vi "isEnd.vi"(10 "pos":i32[][](array[numeric]), 11 "exist":i32[][](array[numeric])) -> (3 "isEnd":i16)   [LabVIEW 2022 SP3, in "subvis.lvlib"]
uses:
  subvis.lvlib
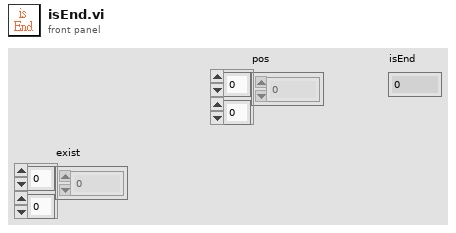
[diagram p1: front panel]
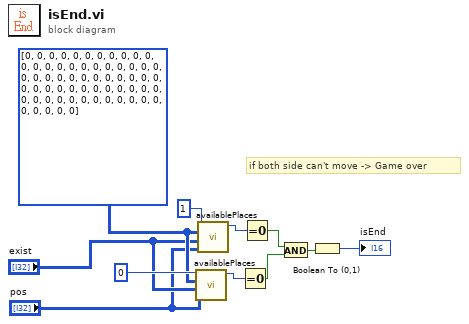
[diagram p0: block diagram]
diagram:
  w4 = i32[][] [[0, 0, 0, 0, 0, 0, 0, 0], [0, 0, 0, 0, 0, 0, 0, 0], [0, 0, 0, 0, 0, 0, 0, 0], [0, 0, 0, 0, 0, 0, 0, 0], [0, 0, 0, 0, 0, 0, 0, 0], [0, 0, 0, 0, 0, 0, 0, 0], [0, 0, 0, 0, 0, 0, 0, 0], [0, 0, 0, 0, 0, 0, 0, 0]] ("availables")
  # "if both side can't move -> Game over"
  n1 = call "availablePlaces.vi"("pos"="pos", "exist"="exist", "available"=w4, "redTurn"=u8 0 ("!redTurn")) -> ("count"=w10:i32)  [unwired: 4 in, 3 out]
  n2 = call "availablePlaces.vi"("pos"="pos", "exist"="exist", "available"=w4, "redTurn"=u8 1) -> ("count"=w11:i32)  [unwired: 4 in, 3 out]
  n3 = Equal To 0?(x=w10) -> (x = 0?=w8:bool)
  n4 = Equal To 0?(x=w11) -> (x = 0?=w9:bool)
  n5 = And(x=w9, y=w8) -> (x .and. y?=w7:bool)
  n6 = Boolean To (0,1)(Boolean=w7) -> (0, 1=→"isEnd":i16)
